vi "Is Refnum.vi"(10 "Self":refnum<data-value>) -> (2 "Error":errorcluster)   [LabVIEW 2021, in "jettl.lvlib" / "jettl Queue Actor.lvlib" / "jettl Queue Actor.lvclass"]
uses:
  jettl Queue Actor.lvclass
  Actor/Msg/Msg.lvclass
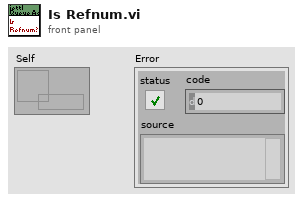
[diagram p1: front panel]
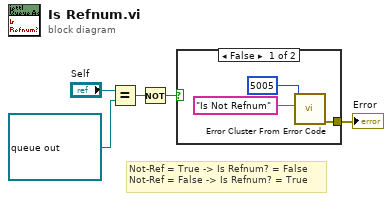
[diagram p0: block diagram]
diagram:
  # "Not-Ref = True -> Is Refnum? = False\nNot-Ref = False -> Is Refnum? = True"
  n1 = Equal?(x="Self", y=refnum<data-value> refnum ("Self")) -> (x = y?=w3:bool)
  n2 = Not(x=w3) -> (.not. x?=w2:bool)
  n3 = case shown="False" w2 {
    tunnel: [w8 _] -> w1
    frame False {
      n4 = call <vilib>:"Error Cluster From Error Code.vi"("error message (\"\")"="Is Not Refnum" ("error message (\"\")"), "error code (0)"=5005) -> ("error out"=w8:errorcluster)  [unwired: 7 in]
    }
    frame True {
    }
  }
  "Error" <- w1
